vi "get_config_cluster.vi"(8 "error in (no error)":errorcluster, 11 "GenericPlugin in":refnum<class "TraceProcessorDL090628DSS.lvclass">) -> (0 "error out":errorcluster, 2 "config cluster (variant)":variant, 3 "GenericPlugin out":refnum<class "TraceProcessorDL090628DSS.lvclass">)   [LabVIEW 2010, in "TraceProcessorDL090628DSS.lvclass"]
uses:
  TraceProcessorDL090628DSS.lvclass
  TraceProcessorDL090628DSS.lvclass/TraceProcessorDL090628DSS.ctl
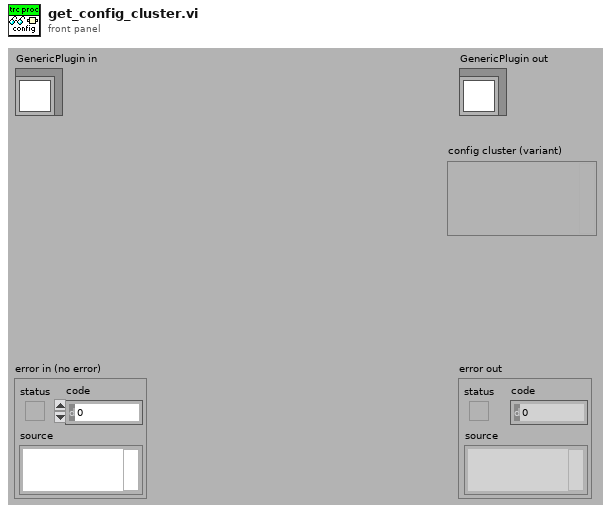
[diagram p1: front panel]
types:
  T1 = typedef "TraceProcessorDL090628DSS.lvclass/config_data_cluster.ctl" = cluster{"baseline sampling pixels":i32}
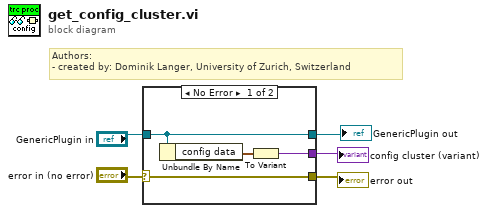
[diagram p0: block diagram]
diagram:
  # "Authors: \n- created by: Dominik Langer, University of Zurich, Switzerland"
  n1 = case shown="No Error" "error in (no error)" {
    selector: "error in (no error)" -> [w6 w10]
    tunnel: "GenericPlugin in" -> [w9 w11]
    tunnel: [w9 w11] -> w2
    tunnel: [w7 _] -> w3
    tunnel: [w6 w10] -> w1
    frame No Error {
      n2 = Unbundle By Name(w9) -> ("config data"=w8:T1)
      n3 = To Variant(anything=w8) -> (Variant=w7:variant)
    }
    frame Error {
    }
  }
  "error out" <- w1
  "GenericPlugin out" <- w2
  "config cluster (variant)" <- w3
